vi "main_QMH_remake.vi"() -> ()   [LabVIEW 2015]
uses:
  Type Definitions/DLTS_input_parameters.ctl
  Type Definitions/state_commands.ctl
panel:
  in  "Settings Button":bool
  out "error out":errorcluster
  out "Bias, pulse and boonton Cluster 2":T1 {"Delay time (ms)" format="%#_4p"; "# Windows" format="%#_4p"; "min window length (ms)" format="%#_4p"; "Pulse width (ms)" format="%#_4p"}
  out "Indicators Cluster":T2 {"Transient length (s)" format="%#_4p"}
  in  "DLTS_input_parameters":T3 {"Delay time (ms)" format="%#_4p"; "# Windows" format="%#_4p"; "min window length (ms)" format="%#_4p"; "Pulse width (ms)" format="%#_4p"}
  in  "File Location":path
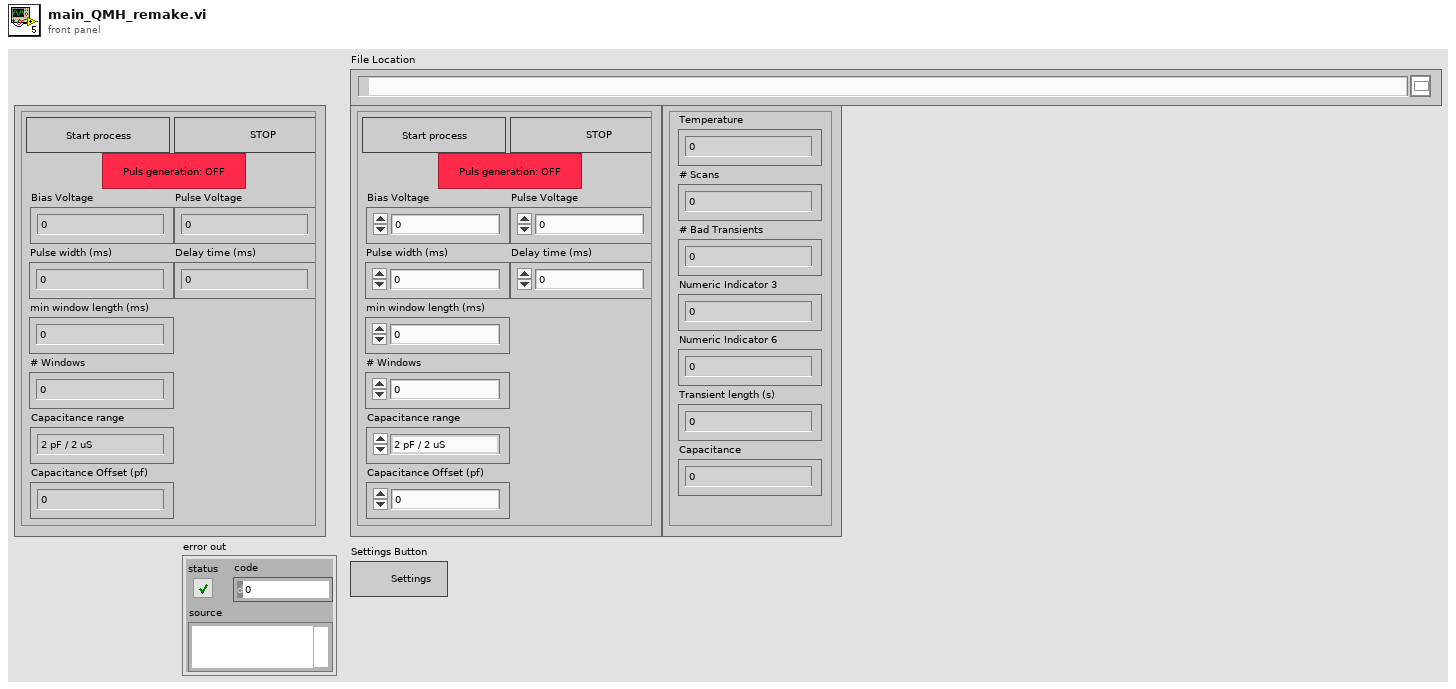
[diagram p1: front panel]
types:
  T1 = cluster{"Pulse Voltage":dbl, "Bias Voltage":dbl, "Pulse ON/OFF":bool, "Pulse width (ms)":dbl, "min window length (ms)":dbl, "# Windows":dbl, "Delay time (ms)":dbl, "Capacitance range":enum16{"2 pF / 2 uS", "20 pF / 20 uS", "200 pF / 200 uS", "2000 pF / 2000 uS"}, "Capacitance Offset (pf)":dbl, "Start process":bool, "STOP":bool}
  T2 = cluster{"Temperature":dbl, "# Bad Transients":dbl, "Numeric Indicator 3":dbl, "# Scans":dbl, "Numeric Indicator 6":dbl, "Transient length (s)":dbl, "Capacitance ":dbl}
  T3 = typedef "DLTS_input_parameters.ctl" = cluster{"Pulse Voltage":dbl, "Bias Voltage":dbl, "Pulse ON/OFF":bool, "Pulse width (ms)":dbl, "min window length (ms)":dbl, "# Windows":dbl, "Delay time (ms)":dbl, "Capacitance range":enum16{"2 pF / 2 uS", "20 pF / 20 uS", "200 pF / 200 uS", "2000 pF / 2000 uS"}, "Capacitance Offset (pf)":dbl, "Start process":bool, "STOP":bool}
  T4 = typedef "state_commands.ctl" = enum16{"Initialize", "Update", "Stop", "Settings"}
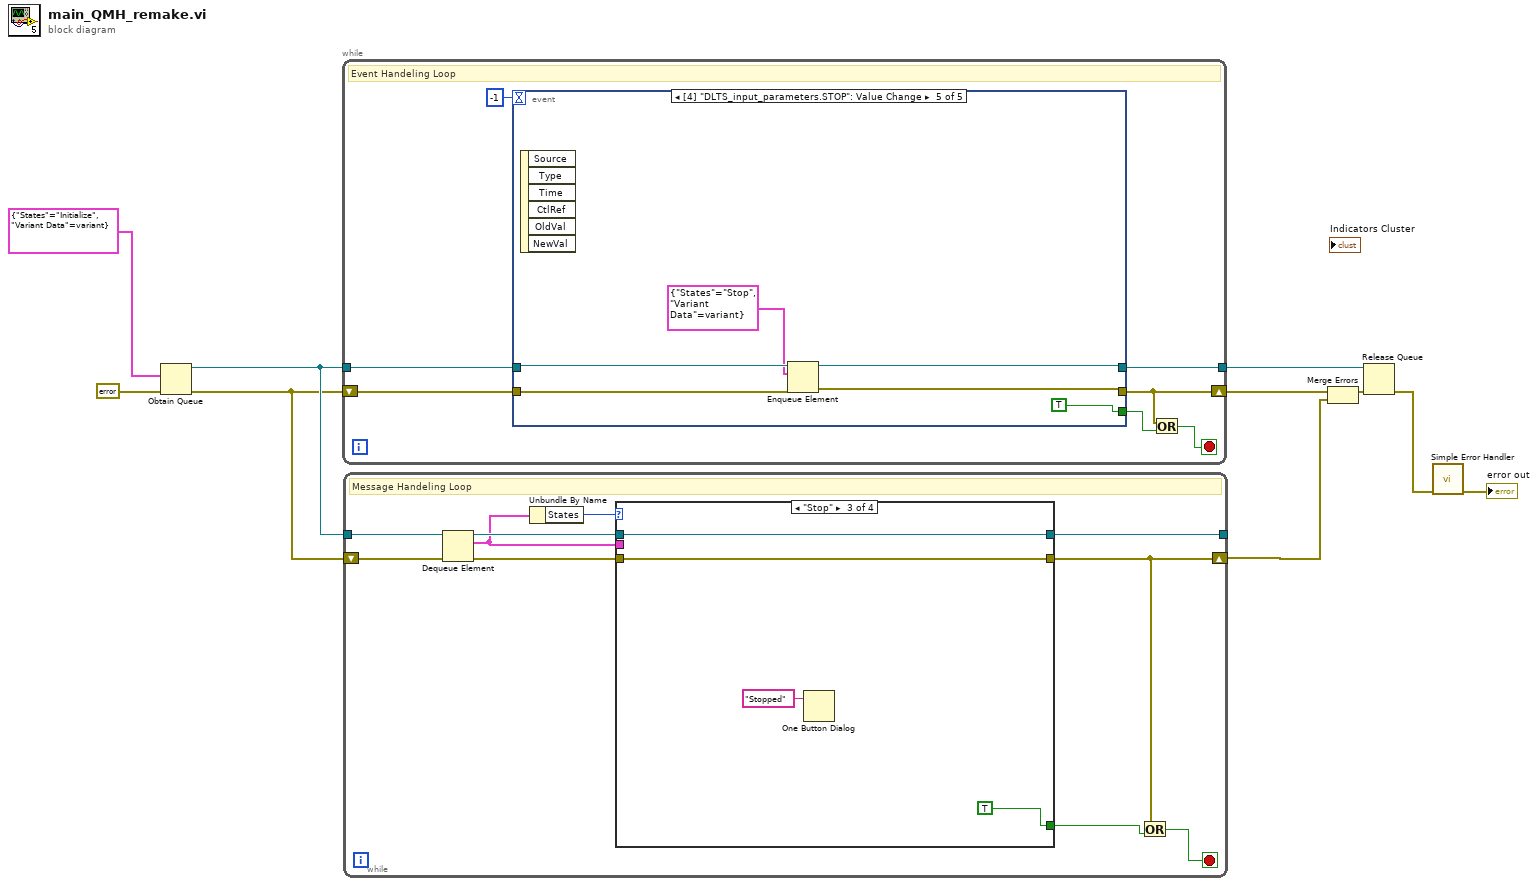
[diagram p0: block diagram]
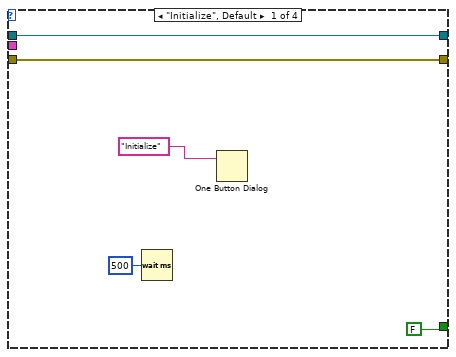
[diagram p2: hidden frame]
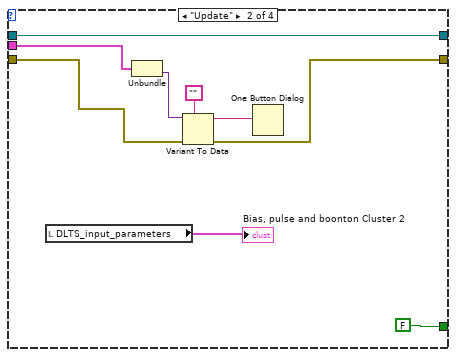
[diagram p3: hidden frame]
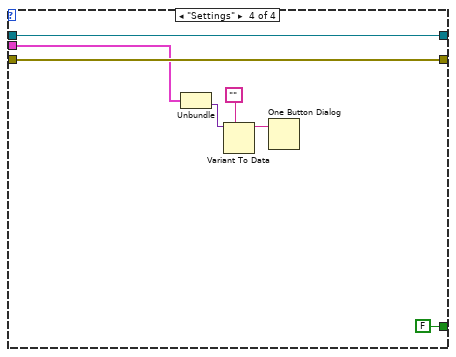
[diagram p4: hidden frame]
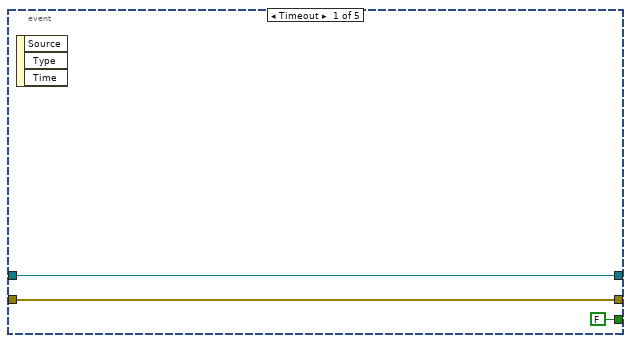
[diagram p5: hidden frame]
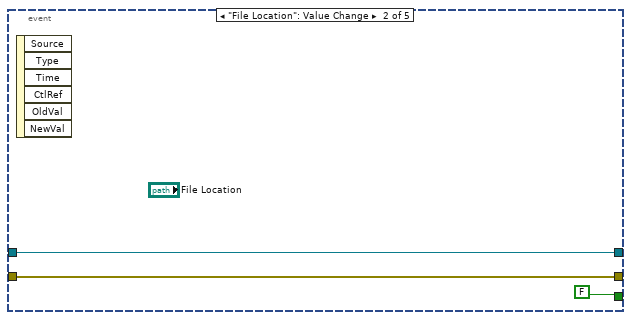
[diagram p6: hidden frame]
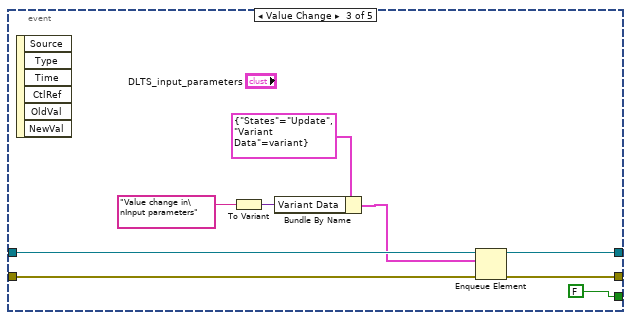
[diagram p7: hidden frame]
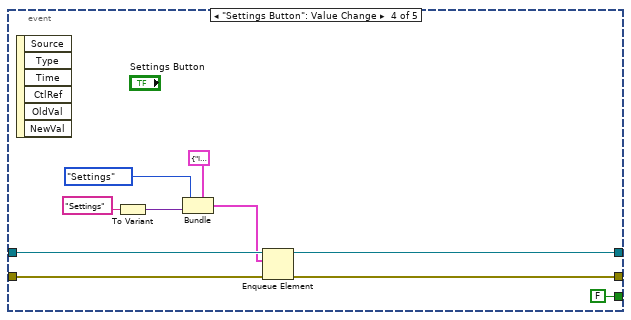
[diagram p8: hidden frame]
diagram:
  n1 = Obtain Queue(element data type=cluster{"States":T4, "Variant Data":variant} {"States"=enum."Initialize", "Variant Data"=variant}, error in (no error)=errorcluster {"status"=FALSE, "code"=0, "source"=""}) -> (queue out=w8:refnum<queue>, error out=w7:errorcluster)  [unwired: 3 in, 1 out]
  n2 = while {
    shift-right: [w12] -> w3
    shift-left: w7 -> [w14]
    tunnel: w8 -> [w15]
    tunnel: [w17] -> w4
    stop <- w13 stop-if-true
    # "Event Handeling Loop"
    n3 = event shown="[4] \"DLTS_input_parameters.STOP\": Value Change" {
      selector: _ -> [_ _ _ _ _]
      dyn-events: _ -> [_ _ _ _ _]
      timeout: -1 -> [_ _ _ _ _]
      tunnel: [FALSE FALSE FALSE FALSE TRUE] -> w11
      tunnel: w15 -> [w19 w21 w32 w42 w47]
      tunnel: w14 -> [w20 w22 w31 w34 w46]
      tunnel: [w20 w22 w29 w35 w43] -> w12
      tunnel: [w19 w21 w30 w41 w44] -> w17
      event Timeout {
        n4 = event-data() -> ()  [unwired: 1 in, 3 out]
      }
      event "File Location": Value Change {
        n5 = event-data() -> ()  [unwired: 1 in, 6 out]
      }
      event Value Change {
        n6 = event-data() -> ()  [unwired: 1 in, 6 out]
        n7 = To Variant(anything="Value change in\nInput parameters") -> (Variant=w25:variant)
        n8 = Bundle By Name(cluster=cluster{"States":T4, "Variant Data":variant} {"States"=enum."Update", "Variant Data"=variant}, "Variant Data"=w25) -> (w27:cluster{"States":T4, "Variant Data":variant})
        n9 = Enqueue Element(queue=w32, element=w27, error in (no error)=w31) -> (queue out=w30:refnum<queue>, error out=w29:errorcluster)  [unwired: 1 in, 1 out]
      }
      event "Settings Button": Value Change {
        n10 = event-data() -> ()  [unwired: 1 in, 6 out]
        n11 = To Variant(anything="Settings") -> (Variant=w39:variant)
        n12 = Bundle(cluster=cluster{"Enum":T4, variant} {"Enum"=enum."Initialize", variant}, "Enum"=state_commands."Settings", w39) -> (w37:cluster{"Enum":T4, variant})
        n13 = Enqueue Element(queue=w42, element=w37, error in (no error)=w34) -> (queue out=w41:refnum<queue>, error out=w35:errorcluster)  [unwired: 1 in, 1 out]
      }
      event Value Change {
        n14 = event-data() -> ()  [unwired: 1 in, 6 out]
        n15 = Enqueue Element(queue=w47, element=cluster{"States":T4, "Variant Data":variant} {"States"=enum."Stop", "Variant Data"=variant}, error in (no error)=w46) -> (queue out=w44:refnum<queue>, error out=w43:errorcluster)  [unwired: 1 in, 1 out]
      }
    }
    n16 = Or(x=w12, y=w11) -> (x .or. y?=w13:bool)
  }
  n17 = while {
    tunnel: w8 -> [w58]
    tunnel: [w54] -> _
    shift-right: [w49] -> w1
    shift-left: w7 -> [w53]
    stop <- w51 stop-if-true
    # "Message Handeling Loop"
    n18 = Dequeue Element(queue=w58, error in (no error)=w53) -> (queue out=w56:refnum<queue>, element=w52:cluster{"States":T4, "Variant Data":variant}, error out=w55:errorcluster)  [unwired: 1 in, 1 out]
    n19 = Unbundle By Name(w52) -> ("States"=w57:T4)
    n20 = case shown="\"Stop\"" w57 {
      tunnel: w56 -> [w62 w66 w76 w79]
      tunnel: w55 -> [w63 w67 w75 w78]
      tunnel: [w63 w69 w75 w78] -> w49
      tunnel: [w62 w66 w76 w79] -> w54
      tunnel: [FALSE FALSE TRUE FALSE ("true")] -> w50
      tunnel: w52 -> [_ w68 _ w77]
      frame "Initialize", Default {
        n21 = Wait (ms)(milliseconds to wait=u32 500) -> ()  [unwired: 1 out]
        n22 = One Button Dialog(message="Initialize") -> ()  [unwired: 1 in, 1 out]
      }
      frame "Update" {
        n23 = local read "DLTS_input_parameters"() -> (→"Bias, pulse and boonton Cluster 2":T3)
        n24 = Unbundle(w68) -> ("Variant Data"=w71:variant)  [unwired: 1 out]
        n25 = Variant To Data(error in=w67, type="", Variant=w71) -> (data=w70:string, error out=w69:errorcluster)
        n26 = One Button Dialog(message=w70) -> ()  [unwired: 1 in, 1 out]
      }
      frame "Stop" {
        n27 = One Button Dialog(message="Stopped") -> ()  [unwired: 1 in, 1 out]
      }
      frame "Settings" {
        n28 = Unbundle(w77) -> ("Variant Data"=w83:variant)  [unwired: 1 out]
        n29 = Variant To Data(type="", Variant=w83) -> (data=w81:string)  [unwired: 1 in, 1 out]
        n30 = One Button Dialog(message=w81) -> ()  [unwired: 1 in, 1 out]
      }
    }
    n31 = Or(x=w49, y=w50) -> (x .or. y?=w51:bool)
  }
  n32 = Merge Errors(w3, w1) -> (w2:errorcluster)
  n33 = Release Queue(queue=w4, error in (no error)=w2) -> (error out=w5:errorcluster)  [unwired: 1 in, 2 out]
  n34 = call <vilib>:"Simple Error Handler.vi"("error in (no error)"=w5) -> ("error out"=→"error out":errorcluster)  [unwired: 4 in, 4 out]
